vi "RunProgram.vi"(7 "numParams":i32, 8 "error in":errorcluster, 10 "params":string[](array[string]), 11 "programName":string) -> (0 "error out":errorcluster)   [LabVIEW 2013]
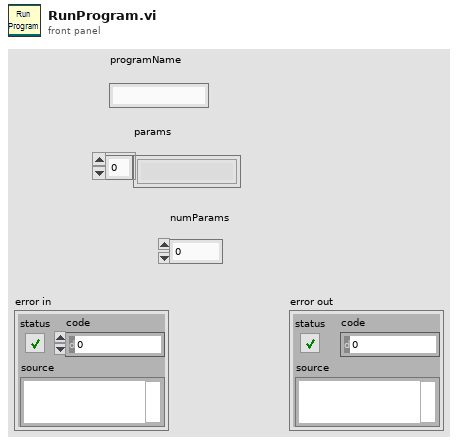
[diagram p1: front panel]
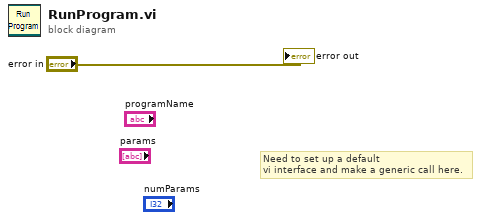
[diagram p0: block diagram]
diagram:
  # "Need to set up a default \nvi interface and make a generic call here."
  "error out" <- "error in"
